vi "SetSelectRowColor(List).vi"(9 "OthersRow":u32(colorbox)=16448250, 10 "SelectRow":u32(colorbox)=12369084, 11 "List输入":refnum<vi>) -> ()   [LabVIEW 2018]
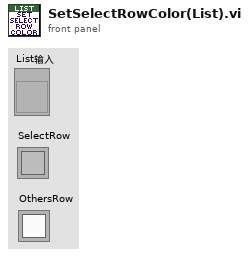
[diagram p1: front panel]
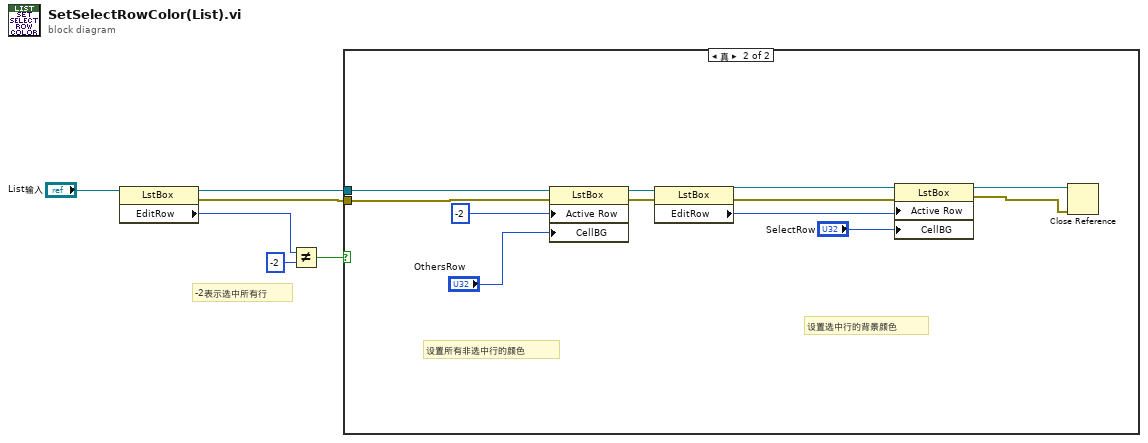
[diagram p0: block diagram]
diagram:
  # "-2表示选中所有行"
  n1 = property class="LstBox"(reference="List输入") -> (reference out=w5:refnum<vi>, error out=w2:errorcluster, "EditRow"=w1:i32)  [unwired: 1 in]
  n2 = Not Equal?(x=w1, y=-2) -> (x != y?=w3:bool)
  n3 = case shown="真" w3 {
    tunnel: w5 -> [_ w14]
    tunnel: w2 -> [_ w13]
    frame False {
    }
    frame True {
      # "设置选中行的背景颜色"
      # "设置所有非选中行的颜色"
      n4 = property class="LstBox"(reference=w14, error in=w13, "Active Row"=-2, "CellBG"="OthersRow") -> (reference out=w12:refnum<vi>, error out=w11:errorcluster)
      n5 = property class="LstBox"(reference=w12, error in=w11) -> (reference out=w18:refnum<vi>, error out=w17:errorcluster, "EditRow"=w8:i32)
      n6 = property class="LstBox"(reference=w18, error in=w17, "Active Row"=w8, "CellBG"="SelectRow") -> (reference out=w16:refnum<vi>, error out=w15:errorcluster)
      n7 = Close Reference(reference=w16, error in (no error)=w15) -> ()  [unwired: 1 out]
    }
  }
